vi "CreateFolder.vi"(0 "DataLogger in":refnum<class "DataLogger.lvclass">, 5 "Save Path":path, 7 "File suffix":string, 9 "StreamToDisk?":bool, 11 "error in (no error)":errorcluster, 12 "SnapShot?":bool) -> (4 "DataLogger out":refnum<class "DataLogger.lvclass">, 6 "Saving Path":path, 8 "Stream Saving Path":path, 10 "Snap Shot Path":path, 15 "error out":errorcluster)   [LabVIEW 2020, in "DataLogger.lvlib" / "DataLogger.lvclass"]
uses:
  DataLogger.lvclass
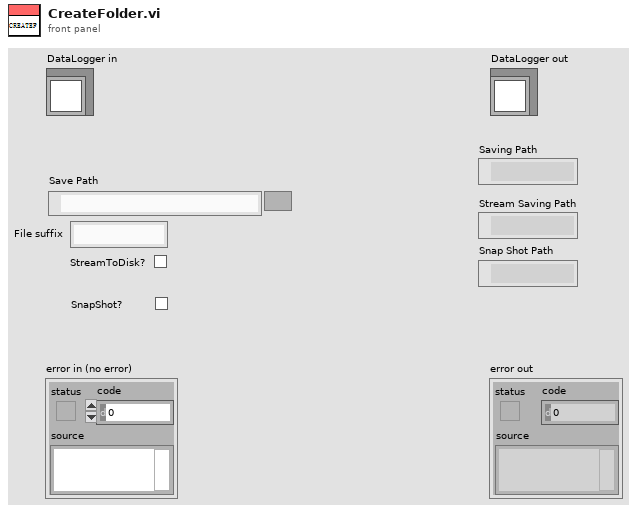
[diagram p1: front panel]
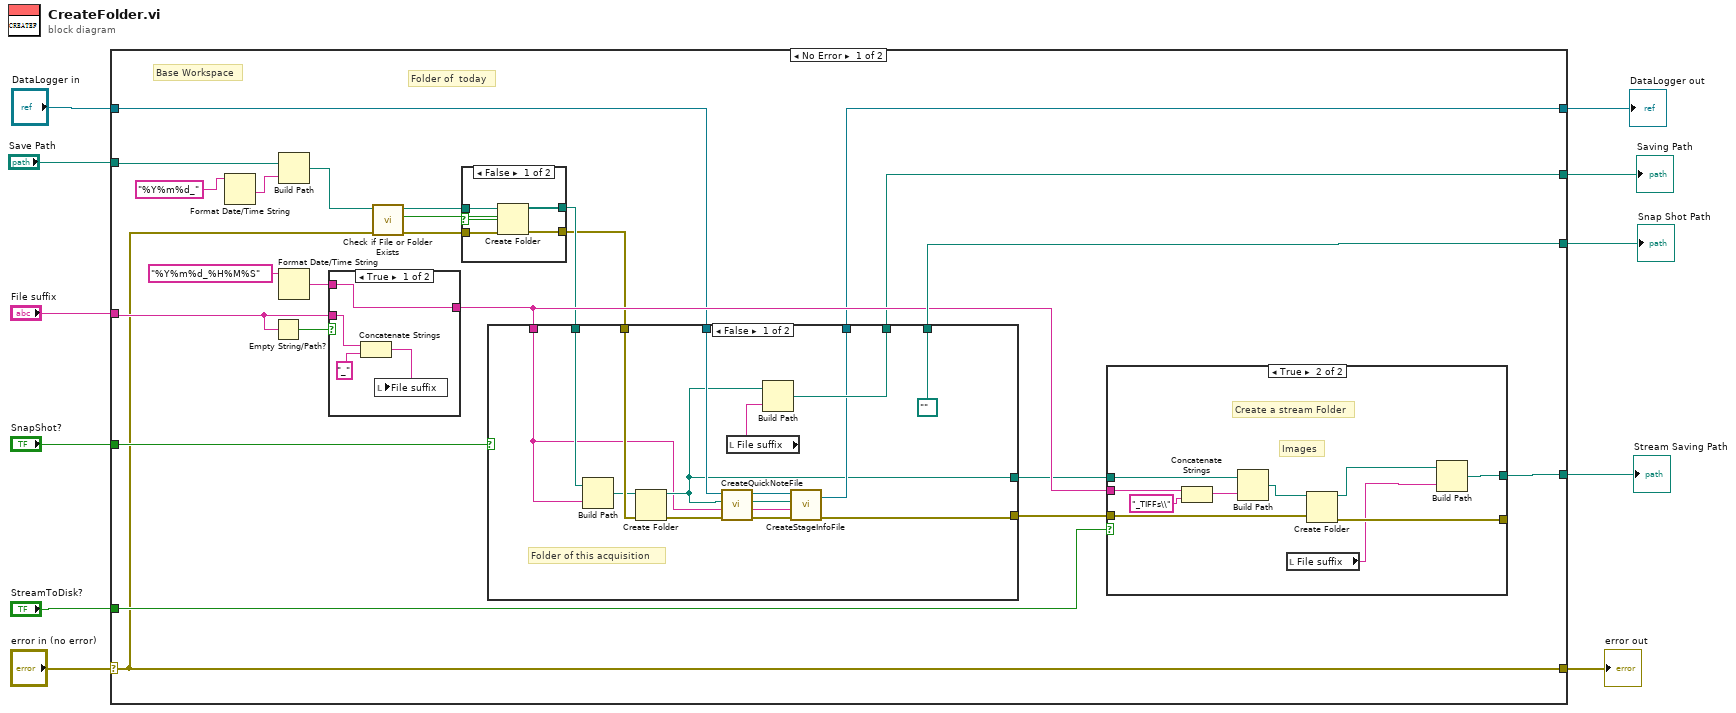
[diagram p0: block diagram]
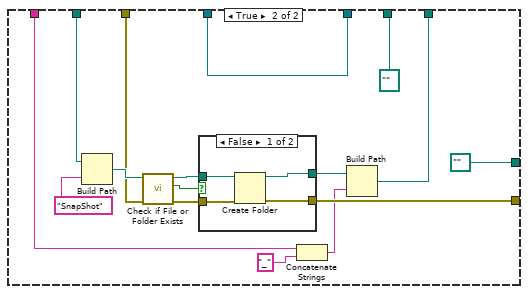
[diagram p2: hidden frame]
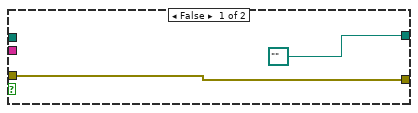
[diagram p4: hidden frame]
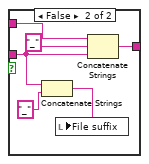
[diagram p5: hidden frame]
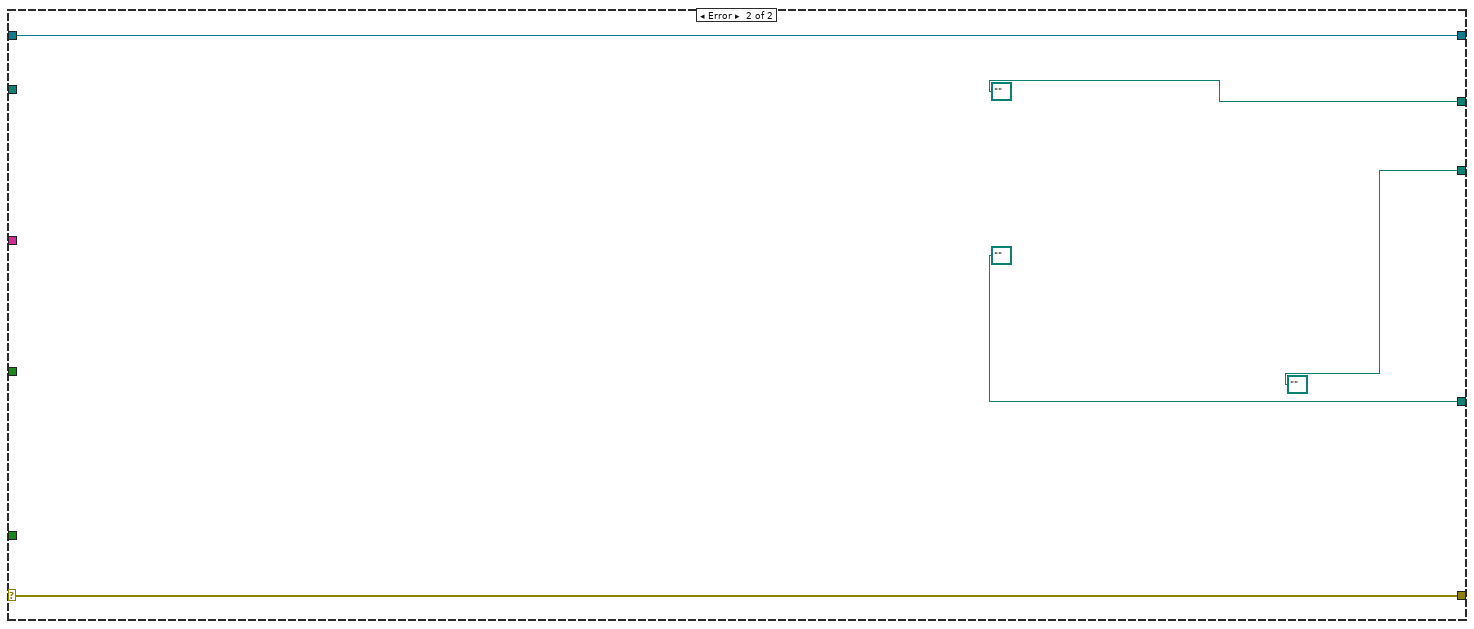
[diagram p7: hidden frame]
diagram:
  n1 = case shown="No Error" "error in (no error)" {
    selector: "error in (no error)" -> [w12 w106]
    tunnel: [w12 w106] -> w4
    tunnel: [w15 w105] -> w1
    tunnel: "DataLogger in" -> [w16 w105]
    tunnel: "Save Path" -> [w27 _]
    tunnel: "File suffix" -> [w14 _]
    tunnel: "StreamToDisk?" -> [w26 _]
    tunnel: [w25 path "" ("created path")] -> w5
    tunnel: [w17 path "" ("created path")] -> w2
    tunnel: "SnapShot?" -> [w24 _]
    tunnel: [w23 path "" ("appended path")] -> w3
    frame No Error {
      # "Base Workspace"
      # "Folder of  today"
      n2 = Format Date/Time String(time format string (%c)="%Y%m%d_") -> (date/time string=w30:string)  [unwired: 2 in]
      n3 = Empty String/Path?(string/path=w14) -> (empty?=w13:bool)
      n4 = Build Path(base path=w27, name or relative path=w30) -> (appended path=w31:path)
      n5 = Format Date/Time String(time format string (%c)="%Y%m%d_%H%M%S") -> (date/time string=w35:string)  [unwired: 2 in]
      n6 = case shown="True" w13 {
        tunnel: w35 -> [w89 w95]
        tunnel: w14 -> [w86 w92]
        tunnel: [w89 w94] -> w22
        frame True {
          n7 = Concatenate Strings(w86, "_" ("string")) -> (w88:string)
          n8 = local write "File suffix"(w88) -> ()
        }
        frame False {
          n9 = Concatenate Strings(w92, "_" ("string")) -> (w90:string)
          n10 = local write "File suffix"(w90) -> ()
          n11 = Concatenate Strings(w95, "_" ("string"), w92) -> (w94:string)
        }
      }
      n12 = call <vilib>:"Check if File or Folder Exists.vi"("error in (no error)"=w12, "path"=w31) -> ("error out"=w34:errorcluster, "file or folder exists?"=w32:bool, "dup path"=w33:path)  [unwired: 7 in]
      n13 = case shown="False" w32 {
        tunnel: w33 -> [w99 w101]
        tunnel: [w98 w100] -> w20
        tunnel: [w97 w101] -> w21
        tunnel: w34 -> [w96 w100]
        frame False {
          n14 = Create Folder(path (use dialog)=w99, error in=w96) -> (created path=w97:path, error out=w98:errorcluster)  [unwired: 1 in, 1 out]
        }
        frame True {
        }
      }
      n15 = case shown="False" w24 {
        tunnel: w21 -> [w47 w67]
        tunnel: [path "" ("appended path") w60] -> w23
        tunnel: w22 -> [w39 w54]
        tunnel: w20 -> [w50 w59]
        tunnel: [w43 w58] -> w19
        tunnel: [w40 path "" ("created path")] -> w18
        tunnel: [w46 path "" ("appended path")] -> w17
        tunnel: w16 -> [w44 w55]
        tunnel: [w41 w55] -> w15
        frame False {
          # "Folder of this acquisition"
          n16 = Build Path(base path=w47, name or relative path=w39) -> (appended path=w49:path)
          n17 = Create Folder(path (use dialog)=w49, error in=w50) -> (created path=w40:path, error out=w48:errorcluster)  [unwired: 1 in, 1 out]
          n18 = call-dynamic "CreateQuickNoteFile.vi"("error in (no error)"=w48, "String"=w39, "created path"=w40, "DataLogger in"=w44) -> ("error out"=w45:errorcluster, "String dup"=w37:string, "created path dup"=w38:path, "DataLogger out"=w42:refnum<class "DataLogger.lvclass">)  [unwired: 4 in]
          n19 = local read "File suffix"() -> (w36:string)
          n20 = Build Path(base path=w40, name or relative path=w36) -> (appended path=w46:path)
          n21 = call-dynamic "CreateStageInfoFile.vi"("error in (no error)"=w45, "String"=w37, "created path"=w38, "DataLogger in"=w42) -> ("error out"=w43:errorcluster, "DataLogger out"=w41:refnum<class "DataLogger.lvclass">)  [unwired: 4 in, 2 out]
        }
        frame True {
          n22 = Build Path(base path=w67, name or relative path="SnapShot") -> (appended path=w65:path)
          n23 = call <vilib>:"Check if File or Folder Exists.vi"("error in (no error)"=w59, "path"=w65) -> ("error out"=w62:errorcluster, "file or folder exists?"=w64:bool, "dup path"=w63:path)  [unwired: 7 in]
          n24 = case shown="False" w64 {
            tunnel: w63 -> [w71 w73]
            tunnel: [w70 w72] -> w58
            tunnel: [w69 w73] -> w61
            tunnel: w62 -> [w68 w72]
            frame False {
              n25 = Create Folder(path (use dialog)=w71, error in=w68) -> (created path=w69:path, error out=w70:errorcluster)  [unwired: 1 in, 1 out]
            }
            frame True {
            }
          }
          n26 = Concatenate Strings(w54, "_" ("string")) -> (w53:string)
          n27 = Build Path(base path=w61, name or relative path=w53) -> (appended path=w60:path)
        }
      }
      n28 = case shown="True" w26 {
        tunnel: [path "" ("created path") w77] -> w25
        tunnel: w19 -> [w75 w85]
        tunnel: [w75 w84] -> _
        tunnel: w18 -> [_ w83]
        tunnel: w22 -> [_ w81]
        frame False {
        }
        frame True {
          # "Create a stream Folder"
          # "Images"
          n29 = Concatenate Strings(w81, "_TIFFs\\" ("string")) -> (w79:string)
          n30 = Build Path(base path=w83, name or relative path=w79) -> (appended path=w82:path)
          n31 = local read "File suffix"() -> (w76:string)
          n32 = Create Folder(path (use dialog)=w82, error in=w85) -> (created path=w78:path, error out=w84:errorcluster)  [unwired: 1 in, 1 out]
          n33 = Build Path(base path=w78, name or relative path=w76) -> (appended path=w77:path)
        }
      }
    }
    frame Error {
    }
  }
  "error out" <- w4
  "DataLogger out" <- w1
  "Saving Path" <- w2
  "Stream Saving Path" <- w5
  "Snap Shot Path" <- w3
